vi "currentReadingLoop.vi"   [LabVIEW 2018]
uses:
  <vilib>/Platform/TimedLoop/XDataNode/timing_clust.ctl
  <vilib>/Platform/TimedLoop/XDataNode/nitl_modes.ctl
  <vilib>/Platform/TimedLoop/XDataNode/wakeup.ctl
  <userlib>/836-Library/System/TDMS_V2/Support/TDMS_DevRef.ctl
  <userlib>/836-Library/System/TDMS_V2/Support/Logging_Settings.ctl
  <userlib>/836-Library/System/TDMS_V2/Support/Group_FIFO_Config.ctl
  <userlib>/836-Library/System/TDMS_V2/Support/Channel_FIFO_Config.ctl
  <vilib>/Rock Robotics/WPI/ThirdParty/Phoenix-LabVIEW/Motor Controller/Get/CTRE_Phoenix_MotorController_GetOutputCurrent_Enhanced.vi
  <vilib>/platform/TimedLoop/XDataNode/XDataNode.xnode
  <vilib>/Platform/TimedLoop/XDataNode/XDNodeRunTimeDep.lvlib
types:
  T1 = typedef "WPI_MotorControlDeviceRef.ctl" = cluster{"DeviceStatus":errorcluster, "Type":T2, "PWM":cluster{"PWM Channel":T3, "DeadBand":T4}, "CAN":cluster{"Device Number":u8, "SetOutput VI Ref":variant, "GetOutput VI Ref":variant, "Enable VI Ref":variant, "Disable VI Ref":variant, "Data":variant}, "Invert":bool, "DIO PWM":cluster{"PWM \"Enable\" Channel":T3, "DIOChannel":T5, "PWM Rate":dbl}}
  T2 = typedef "WPI_MotorControlType.ctl" = enum16{"PWM", "CAN", "DIO PWM"}
  T3 = typedef "FPGA_DIOPWMChannel.ctl" = enum8{"PWM 0", "PWM 1", "PWM 2", "PWM 3", "PWM 4", "PWM 5", "PWM 6", "PWM 7", "PWM 8", "PWM 9", "PWM MXP 0", "PWM MXP 1", "PWM MXP 2", "PWM MXP 3", "PWM MXP 4", "PWM MXP 5", "PWM MXP 6", "PWM MXP 7", "PWM MXP 8", "PWM MXP 9", "Invalid"}
  T4 = typedef "WPI_PWMDeadband.ctl" = cluster{"Name":string, "maxPositivePwm":i32, "minPositivePwm":i32, "centerPwm":i32, "maxNegativePwm":i32, "minNegativePwm":i32, "angularRange":u16}
  T5 = typedef "FPGA_DIOChannel.ctl" = enum8{"DIO 0", "DIO 1", "DIO 2", "DIO 3", "DIO 4", "DIO 5", "DIO 6", "DIO 7", "DIO 8", "DIO 9", "DIO MXP 0", "DIO MXP 1", "DIO MXP 2", "DIO MXP 3", "DIO MXP 4", "DIO MXP 5", "DIO MXP 6", "DIO MXP 7", "DIO MXP 8", "DIO MXP 9", "DIO MXP 10", "DIO MXP 11", "DIO MXP 12", "DIO MXP 13", "DIO MXP 14", "DIO MXP 15", "SPI Port CS1", "SPI Port CS2", "SPI Port CS3", "SPI Port MISO", "SPI Port MOSI", "Invalid"}
  T6 = typedef "XDNodeRunTimeDep.lvlib/timing_clust.ctl" = cluster{"Expected End [f-1]":u64, "Actual End [f-1]":u64, "Finished Late? [f-1]":bool, "Expected End [i-1]":u64, "Actual End [i-1]":u64, "Finished Late? [i-1]":bool, "Expected Start [i]":u64, "Actual Start [i]":u64, "Expected Start [f]":u64, "Actual Start [f]":u64, "Source Name":string, "Structure Name":string, "Period":i64, "Deadline":i64, "Offset":i64, "Start":i64, "Priority":i32, "Timeout":i32, "Mode":T7, "Wakeup Reason":T8, "Error":errorcluster, "Source Type":string, "Secondary Source Type":string, "Global End Time":u64, "Global Start Time":u64, "Frame Duration":u64, "Iteration Duration":u64, "Assigned CPU":i32, "I/O Scan Engine Mode":u32}
  T7 = typedef "XDNodeRunTimeDep.lvlib/nitl_modes.ctl" = enum32{"No Change", "Process missed periods, maintain original phase", "Discard missed periods, maintain original phase", "Process missed periods, ignore original phase", "Discard missed periods, ignore original phase"}
  T8 = typedef "XDNodeRunTimeDep.lvlib/wakeup.ctl" = enum32{"Normal", "Aborted", "Asynchronous wakeup", "Timing source error", "Timed loop error", "Timeout"}
  T9 = typedef "TDMS_DevRef.ctl" = cluster{"Name":string, "File Ref":refnum<k34>, "Start Time":timestamp, "Logging Settings":T10, "Group FIFO Config":T11[], "Data To Write":refnum<data-value>, "semaphore":T13, "Ref Time Reset":refnum<k4>}
  T10 = typedef "Logging_Settings.ctl" = cluster{"Data Grab Period":dbl, "File Write Period":dbl, "Max Stored Size":dbl, "Burst Size":dbl}
  T11 = typedef "Group_FIFO_Config.ctl" = cluster{"Group":string, "Channels":T12[], "Channel Names":string[]}
  T12 = typedef "Channel_FIFO_Config.ctl" = cluster{"Channel":string, "FIFO":refnum<k33>}
  T13 = typedef "Semaphore RefNum" = refnum<k1>
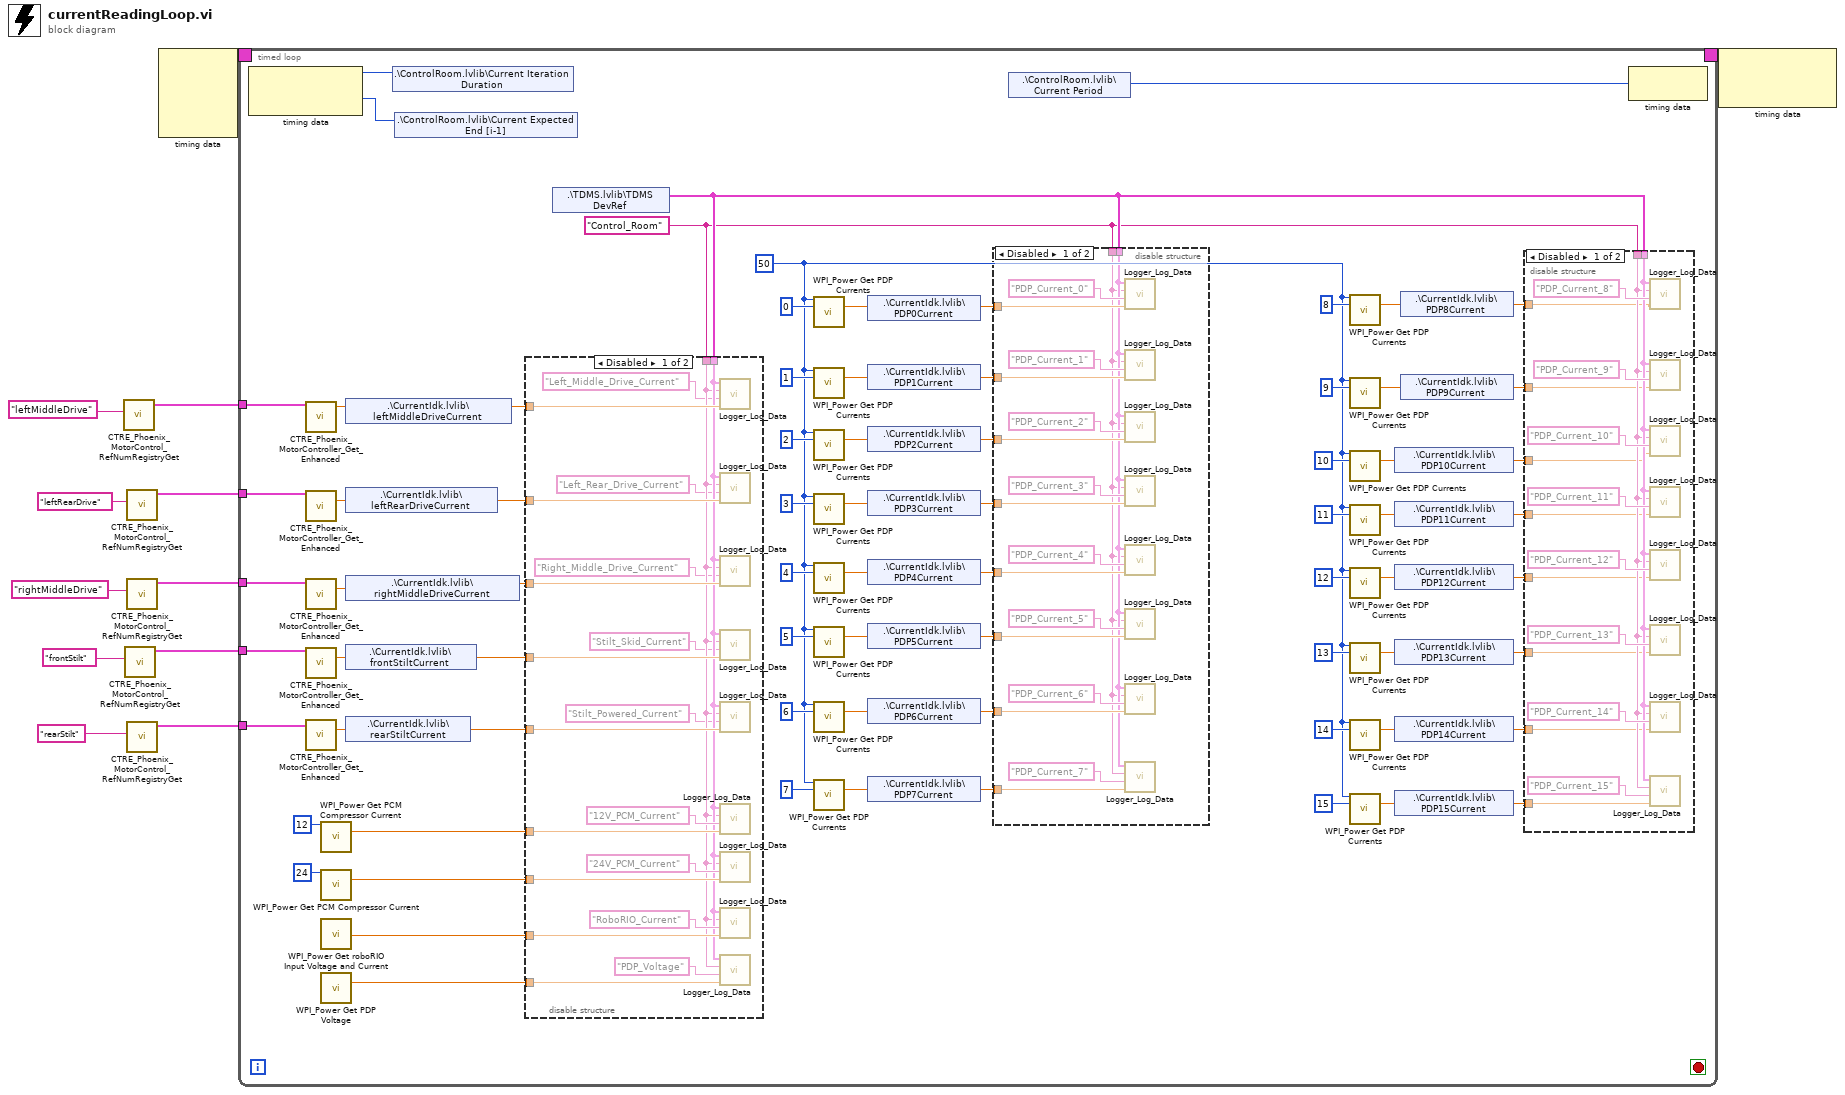
[diagram p0: block diagram]
diagram:
  n1 = call <vilib>:"CTRE_Phoenix_MotorControl_RefNumRegistryGet.vi"("refnum name"="leftMiddleDrive") -> ("PhoenixMotorControlDevRef"=w4:T1)  [unwired: 9 in, 1 out]
  n2 = call <vilib>:"CTRE_Phoenix_MotorControl_RefNumRegistryGet.vi"("refnum name"="frontStilt") -> ("PhoenixMotorControlDevRef"=w6:T1)  [unwired: 9 in, 1 out]
  n3 = call <vilib>:"CTRE_Phoenix_MotorControl_RefNumRegistryGet.vi"("refnum name"="leftRearDrive") -> ("PhoenixMotorControlDevRef"=w5:T1)  [unwired: 9 in, 1 out]
  n4 = call <vilib>:"CTRE_Phoenix_MotorControl_RefNumRegistryGet.vi"("refnum name"="rightMiddleDrive") -> ("PhoenixMotorControlDevRef"=w1:T1)  [unwired: 9 in, 1 out]
  n5 = call <vilib>:"CTRE_Phoenix_MotorControl_RefNumRegistryGet.vi"("refnum name"="rearStilt") -> ("PhoenixMotorControlDevRef"=w7:T1)  [unwired: 9 in, 1 out]
  n6 = node-c288() -> (w9:T6)  [unwired: 4 in]
  n7 = timed-loop {
    timing: w9 -> [_]
    timing-out: [_] -> w8
    tunnel: w7 -> [w64]
    tunnel: w6 -> [w63]
    tunnel: w5 -> [w62]
    tunnel: w4 -> [w61]
    tunnel: w1 -> [w60]
    stop <- _ stop-if-true
    w13 = "Control_Room" ("Group")
    w42 = u8 50 ("Power Distribution Panel (0)")
    n8 = node-c288() -> (w66:i64, w65:i64)  [unwired: 1 in]
    n9 = call-poly <vilib>:"CTRE_Phoenix_MotorController_Get_Enhanced.vi"("PhoenixMotorControlDevRef"=w61) -> ("Output Current"=w41:dbl)  [unwired: 12 in, 2 out]
    n10 = call-poly <vilib>:"CTRE_Phoenix_MotorController_Get_Enhanced.vi"("PhoenixMotorControlDevRef"=w62) -> ("Output Current"=w40:dbl)  [unwired: 12 in, 2 out]
    n11 = call-poly <vilib>:"CTRE_Phoenix_MotorController_Get_Enhanced.vi"("PhoenixMotorControlDevRef"=w60) -> ("Output Current"=w37:dbl)  [unwired: 12 in, 2 out]
    n12 = call-poly <vilib>:"CTRE_Phoenix_MotorController_Get_Enhanced.vi"("PhoenixMotorControlDevRef"=w63) -> ("Output Current"=w38:dbl)  [unwired: 12 in, 2 out]
    n13 = call-poly <vilib>:"CTRE_Phoenix_MotorController_Get_Enhanced.vi"("PhoenixMotorControlDevRef"=w64) -> ("Output Current"=w39:dbl)  [unwired: 12 in, 2 out]
    n14 = call <vilib>:"WPI_Power Get PCM Compressor Current.vi"("Pneumatics Control Module (0)"=u8 12) -> ("current (A)"=w18:dbl)  [unwired: 13 in, 1 out]
    n15 = call <vilib>:"WPI_Power Get PCM Compressor Current.vi"("Pneumatics Control Module (0)"=u8 24) -> ("current (A)"=w17:dbl)  [unwired: 13 in, 1 out]
    n16 = call <vilib>:"WPI_Power Get roboRIO Input Voltage and Current.vi"() -> ("roboRIO input current (A)"=w16:dbl)  [unwired: 13 in, 2 out]
    n17 = call <vilib>:"WPI_Power Get PDP Voltage.vi"() -> ("voltage (V)"=w15:dbl)  [unwired: 14 in, 1 out]
    n18 = shared-variable ".\\CurrentIdk.lvlib\\leftMiddleDriveCurrent"(w41) -> ()  [unwired: 1 in, 1 out]
    n19 = shared-variable ".\\CurrentIdk.lvlib\\leftRearDriveCurrent"(w40) -> ()  [unwired: 1 in, 1 out]
    n20 = shared-variable ".\\CurrentIdk.lvlib\\rightMiddleDriveCurrent"(w37) -> ()  [unwired: 1 in, 1 out]
    n21 = shared-variable ".\\CurrentIdk.lvlib\\frontStiltCurrent"(w38) -> ()  [unwired: 1 in, 1 out]
    n22 = shared-variable ".\\CurrentIdk.lvlib\\rearStiltCurrent"(w39) -> ()  [unwired: 1 in, 1 out]
    n23 = shared-variable ".\\ControlRoom.lvlib\\Current Iteration Duration"(w66) -> ()  [unwired: 1 in, 1 out]
    n24 = shared-variable ".\\ControlRoom.lvlib\\Current Expected End [i-1]"(w65) -> ()  [unwired: 1 in, 1 out]
    n25 = shared-variable ".\\TDMS.lvlib\\TDMS DevRef"() -> (w14:T9)  [unwired: 1 in, 1 out]
    n26 = disable-structure shown="Disabled" {
      disable-tunnel: w41 -> [w86 _]
      disable-tunnel: w40 -> [w85 _]
      disable-tunnel: w39 -> [w84 _]
      disable-tunnel: w38 -> [w83 _]
      disable-tunnel: w37 -> [w82 _]
      disable-tunnel: w18 -> [w80 _]
      disable-tunnel: w17 -> [w76 _]
      disable-tunnel: w16 -> [w75 _]
      disable-tunnel: w15 -> [w74 _]
      disable-tunnel: w14 -> [w73 _]
      disable-tunnel: w13 -> [w72 _]
      frame Disabled {
        n27 = call <userlib>:"Logger_Log_Data.vi"("Data"=w86, "Channel"="Left_Middle_Drive_Current", "Group"=w72, "TDMS DevRef"=w73) -> ()  [unwired: 7 in, 1 out]
        n28 = call <userlib>:"Logger_Log_Data.vi"("Data"=w85, "Channel"="Left_Rear_Drive_Current", "Group"=w72, "TDMS DevRef"=w73) -> ()  [unwired: 7 in, 1 out]
        n29 = call <userlib>:"Logger_Log_Data.vi"("Data"=w82, "Channel"="Right_Middle_Drive_Current", "Group"=w72, "TDMS DevRef"=w73) -> ()  [unwired: 7 in, 1 out]
        n30 = call <userlib>:"Logger_Log_Data.vi"("Data"=w83, "Channel"="Stilt_Skid_Current", "Group"=w72, "TDMS DevRef"=w73) -> ()  [unwired: 7 in, 1 out]
        n31 = call <userlib>:"Logger_Log_Data.vi"("Data"=w84, "Channel"="Stilt_Powered_Current", "Group"=w72, "TDMS DevRef"=w73) -> ()  [unwired: 7 in, 1 out]
        n32 = call <userlib>:"Logger_Log_Data.vi"("Data"=w80, "Channel"="12V_PCM_Current", "Group"=w72, "TDMS DevRef"=w73) -> ()  [unwired: 7 in, 1 out]
        n33 = call <userlib>:"Logger_Log_Data.vi"("Data"=w76, "Channel"="24V_PCM_Current", "Group"=w72, "TDMS DevRef"=w73) -> ()  [unwired: 7 in, 1 out]
        n34 = call <userlib>:"Logger_Log_Data.vi"("Data"=w75, "Channel"="RoboRIO_Current", "Group"=w72, "TDMS DevRef"=w73) -> ()  [unwired: 7 in, 1 out]
        n35 = call <userlib>:"Logger_Log_Data.vi"("Data"=w74, "Channel"="PDP_Voltage", "Group"=w72, "TDMS DevRef"=w73) -> ()  [unwired: 7 in, 1 out]
      }
      frame Enabled {
      }
    }
    n36 = call <vilib>:"WPI_Power Get PDP Currents.vi"("Power Distribution Panel (0)"=w42, "PDP Channel"=0) -> ("current (A)"=w36:dbl)  [unwired: 11 in, 2 out]
    n37 = call <vilib>:"WPI_Power Get PDP Currents.vi"("Power Distribution Panel (0)"=w42, "PDP Channel"=1) -> ("current (A)"=w29:dbl)  [unwired: 11 in, 2 out]
    n38 = call <vilib>:"WPI_Power Get PDP Currents.vi"("Power Distribution Panel (0)"=w42, "PDP Channel"=2) -> ("current (A)"=w30:dbl)  [unwired: 11 in, 2 out]
    n39 = call <vilib>:"WPI_Power Get PDP Currents.vi"("Power Distribution Panel (0)"=w42, "PDP Channel"=3) -> ("current (A)"=w31:dbl)  [unwired: 11 in, 2 out]
    n40 = call <vilib>:"WPI_Power Get PDP Currents.vi"("Power Distribution Panel (0)"=w42, "PDP Channel"=4) -> ("current (A)"=w32:dbl)  [unwired: 11 in, 2 out]
    n41 = call <vilib>:"WPI_Power Get PDP Currents.vi"("Power Distribution Panel (0)"=w42, "PDP Channel"=5) -> ("current (A)"=w33:dbl)  [unwired: 11 in, 2 out]
    n42 = call <vilib>:"WPI_Power Get PDP Currents.vi"("Power Distribution Panel (0)"=w42, "PDP Channel"=6) -> ("current (A)"=w34:dbl)  [unwired: 11 in, 2 out]
    n43 = call <vilib>:"WPI_Power Get PDP Currents.vi"("Power Distribution Panel (0)"=w42, "PDP Channel"=7) -> ("current (A)"=w35:dbl)  [unwired: 11 in, 2 out]
    n44 = shared-variable ".\\CurrentIdk.lvlib\\PDP0Current"(w36) -> ()  [unwired: 1 in, 1 out]
    n45 = shared-variable ".\\CurrentIdk.lvlib\\PDP1Current"(w29) -> ()  [unwired: 1 in, 1 out]
    n46 = shared-variable ".\\CurrentIdk.lvlib\\PDP2Current"(w30) -> ()  [unwired: 1 in, 1 out]
    n47 = shared-variable ".\\CurrentIdk.lvlib\\PDP3Current"(w31) -> ()  [unwired: 1 in, 1 out]
    n48 = shared-variable ".\\CurrentIdk.lvlib\\PDP4Current"(w32) -> ()  [unwired: 1 in, 1 out]
    n49 = shared-variable ".\\CurrentIdk.lvlib\\PDP5Current"(w33) -> ()  [unwired: 1 in, 1 out]
    n50 = shared-variable ".\\CurrentIdk.lvlib\\PDP6Current"(w34) -> ()  [unwired: 1 in, 1 out]
    n51 = shared-variable ".\\CurrentIdk.lvlib\\PDP7Current"(w35) -> ()  [unwired: 1 in, 1 out]
    n52 = disable-structure shown="Disabled" {
      disable-tunnel: w36 -> [w121 _]
      disable-tunnel: w35 -> [w113 _]
      disable-tunnel: w34 -> [w112 _]
      disable-tunnel: w33 -> [w111 _]
      disable-tunnel: w32 -> [w110 _]
      disable-tunnel: w31 -> [w109 _]
      disable-tunnel: w30 -> [w108 _]
      disable-tunnel: w29 -> [w107 _]
      disable-tunnel: w14 -> [w106 _]
      disable-tunnel: w13 -> [w105 _]
      frame Disabled {
        n53 = call <userlib>:"Logger_Log_Data.vi"("Data"=w121, "Channel"="PDP_Current_0", "Group"=w105, "TDMS DevRef"=w106) -> ()  [unwired: 7 in, 1 out]
        n54 = call <userlib>:"Logger_Log_Data.vi"("Data"=w107, "Channel"="PDP_Current_1", "Group"=w105, "TDMS DevRef"=w106) -> ()  [unwired: 7 in, 1 out]
        n55 = call <userlib>:"Logger_Log_Data.vi"("Data"=w108, "Channel"="PDP_Current_2", "Group"=w105, "TDMS DevRef"=w106) -> ()  [unwired: 7 in, 1 out]
        n56 = call <userlib>:"Logger_Log_Data.vi"("Data"=w109, "Channel"="PDP_Current_3", "Group"=w105, "TDMS DevRef"=w106) -> ()  [unwired: 7 in, 1 out]
        n57 = call <userlib>:"Logger_Log_Data.vi"("Data"=w110, "Channel"="PDP_Current_4", "Group"=w105, "TDMS DevRef"=w106) -> ()  [unwired: 7 in, 1 out]
        n58 = call <userlib>:"Logger_Log_Data.vi"("Data"=w111, "Channel"="PDP_Current_5", "Group"=w105, "TDMS DevRef"=w106) -> ()  [unwired: 7 in, 1 out]
        n59 = call <userlib>:"Logger_Log_Data.vi"("Data"=w112, "Channel"="PDP_Current_6", "Group"=w105, "TDMS DevRef"=w106) -> ()  [unwired: 7 in, 1 out]
        n60 = call <userlib>:"Logger_Log_Data.vi"("Data"=w113, "Channel"="PDP_Current_7", "Group"=w105, "TDMS DevRef"=w106) -> ()  [unwired: 7 in, 1 out]
      }
      frame Enabled {
      }
    }
    n61 = shared-variable ".\\ControlRoom.lvlib\\Current Period"() -> (w43:i64)  [unwired: 1 in, 1 out]
    n62 = call <vilib>:"WPI_Power Get PDP Currents.vi"("Power Distribution Panel (0)"=w42, "PDP Channel"=8) -> ("current (A)"=w28:dbl)  [unwired: 11 in, 2 out]
    n63 = call <vilib>:"WPI_Power Get PDP Currents.vi"("Power Distribution Panel (0)"=w42, "PDP Channel"=9) -> ("current (A)"=w27:dbl)  [unwired: 11 in, 2 out]
    n64 = call <vilib>:"WPI_Power Get PDP Currents.vi"("Power Distribution Panel (0)"=w42, "PDP Channel"=10) -> ("current (A)"=w26:dbl)  [unwired: 11 in, 2 out]
    n65 = call <vilib>:"WPI_Power Get PDP Currents.vi"("Power Distribution Panel (0)"=w42, "PDP Channel"=11) -> ("current (A)"=w25:dbl)  [unwired: 11 in, 2 out]
    n66 = call <vilib>:"WPI_Power Get PDP Currents.vi"("Power Distribution Panel (0)"=w42, "PDP Channel"=12) -> ("current (A)"=w24:dbl)  [unwired: 11 in, 2 out]
    n67 = call <vilib>:"WPI_Power Get PDP Currents.vi"("Power Distribution Panel (0)"=w42, "PDP Channel"=13) -> ("current (A)"=w23:dbl)  [unwired: 11 in, 2 out]
    n68 = call <vilib>:"WPI_Power Get PDP Currents.vi"("Power Distribution Panel (0)"=w42, "PDP Channel"=14) -> ("current (A)"=w22:dbl)  [unwired: 11 in, 2 out]
    n69 = call <vilib>:"WPI_Power Get PDP Currents.vi"("Power Distribution Panel (0)"=w42, "PDP Channel"=15) -> ("current (A)"=w21:dbl)  [unwired: 11 in, 2 out]
    n70 = shared-variable ".\\CurrentIdk.lvlib\\PDP10Current"(w26) -> ()  [unwired: 1 in, 1 out]
    n71 = shared-variable ".\\CurrentIdk.lvlib\\PDP11Current"(w25) -> ()  [unwired: 1 in, 1 out]
    n72 = shared-variable ".\\CurrentIdk.lvlib\\PDP12Current"(w24) -> ()  [unwired: 1 in, 1 out]
    n73 = shared-variable ".\\CurrentIdk.lvlib\\PDP13Current"(w23) -> ()  [unwired: 1 in, 1 out]
    n74 = shared-variable ".\\CurrentIdk.lvlib\\PDP14Current"(w22) -> ()  [unwired: 1 in, 1 out]
    n75 = shared-variable ".\\CurrentIdk.lvlib\\PDP15Current"(w21) -> ()  [unwired: 1 in, 1 out]
    n76 = shared-variable ".\\CurrentIdk.lvlib\\PDP8Current"(w28) -> ()  [unwired: 1 in, 1 out]
    n77 = shared-variable ".\\CurrentIdk.lvlib\\PDP9Current"(w27) -> ()  [unwired: 1 in, 1 out]
    n78 = disable-structure shown="Disabled" {
      disable-tunnel: w14 -> [w96 _]
      disable-tunnel: w13 -> [w95 _]
      disable-tunnel: w28 -> [w94 _]
      disable-tunnel: w27 -> [w93 _]
      disable-tunnel: w26 -> [w92 _]
      disable-tunnel: w25 -> [w91 _]
      disable-tunnel: w24 -> [w90 _]
      disable-tunnel: w23 -> [w89 _]
      disable-tunnel: w22 -> [w88 _]
      disable-tunnel: w21 -> [w87 _]
      frame Disabled {
        n79 = call <userlib>:"Logger_Log_Data.vi"("Data"=w94, "Channel"="PDP_Current_8", "Group"=w95, "TDMS DevRef"=w96) -> ()  [unwired: 7 in, 1 out]
        n80 = call <userlib>:"Logger_Log_Data.vi"("Data"=w93, "Channel"="PDP_Current_9", "Group"=w95, "TDMS DevRef"=w96) -> ()  [unwired: 7 in, 1 out]
        n81 = call <userlib>:"Logger_Log_Data.vi"("Data"=w92, "Channel"="PDP_Current_10", "Group"=w95, "TDMS DevRef"=w96) -> ()  [unwired: 7 in, 1 out]
        n82 = call <userlib>:"Logger_Log_Data.vi"("Data"=w91, "Channel"="PDP_Current_11", "Group"=w95, "TDMS DevRef"=w96) -> ()  [unwired: 7 in, 1 out]
        n83 = call <userlib>:"Logger_Log_Data.vi"("Data"=w90, "Channel"="PDP_Current_12", "Group"=w95, "TDMS DevRef"=w96) -> ()  [unwired: 7 in, 1 out]
        n84 = call <userlib>:"Logger_Log_Data.vi"("Data"=w89, "Channel"="PDP_Current_13", "Group"=w95, "TDMS DevRef"=w96) -> ()  [unwired: 7 in, 1 out]
        n85 = call <userlib>:"Logger_Log_Data.vi"("Data"=w88, "Channel"="PDP_Current_14", "Group"=w95, "TDMS DevRef"=w96) -> ()  [unwired: 7 in, 1 out]
        n86 = call <userlib>:"Logger_Log_Data.vi"("Data"=w87, "Channel"="PDP_Current_15", "Group"=w95, "TDMS DevRef"=w96) -> ()  [unwired: 7 in, 1 out]
      }
      frame Enabled {
      }
    }
    n87 = node-c288(w43) -> ()  [unwired: 1 out]
  }
  n88 = node-c288(w8) -> ()  [unwired: 2 out]
